vi "WriteSpreadsheet.vi"(0 "2-d array of\nnumbers":dbl[][](array[numeric])) -> ()   [LabVIEW 2023]
doc: "This is a tool that was written to allow users the opportunity to preview the files before they save them into a spreadsheet. The precision can be input and the header can be setup prior to saving the data."
panel:
  in  "invert data":bool
  in  "cancel":bool
  in  "save":bool
  in  "header":string[][](table)=[["User Name", "", "", "", "", "", "", "", "", "", ""], ["Experimental Description", "", "", "", "", "", "", "", "", "", ""], ["Header A (units)", "Header B (u)", "Header C (u)", "Header D (u)", "", "", "", "", "", "", ""]]
  in  "precision":i16=6 caption="input the desired\ndata precision"
  out "spreadsheet":string[][](table)=[["Sunday, January 10, 2010", "", "", "", "", "", "", "", "", "", ""], ["User Name", "", "", "", "", "", "", "", "", "", ""], ["Experimental Description", "", "", "", "", "", "", "", "", "", ""], ["Header A (units)", "Header B (u)", "Header C (u)", "Header D (u)", "", "", "", "", "", "", ""], ["NaN", "NaN", "NaN", "NaN", "", "", "", "", "", "", ""], ["NaN", "NaN", "NaN", "NaN", "", "", "", "", "", "", ""], ["NaN", "NaN", "NaN", "NaN", "", "", "", "", "", "", ""]]
  # "Input File Information and Headers (editable)"
  # "Spread Sheet Viewer (not editable)"
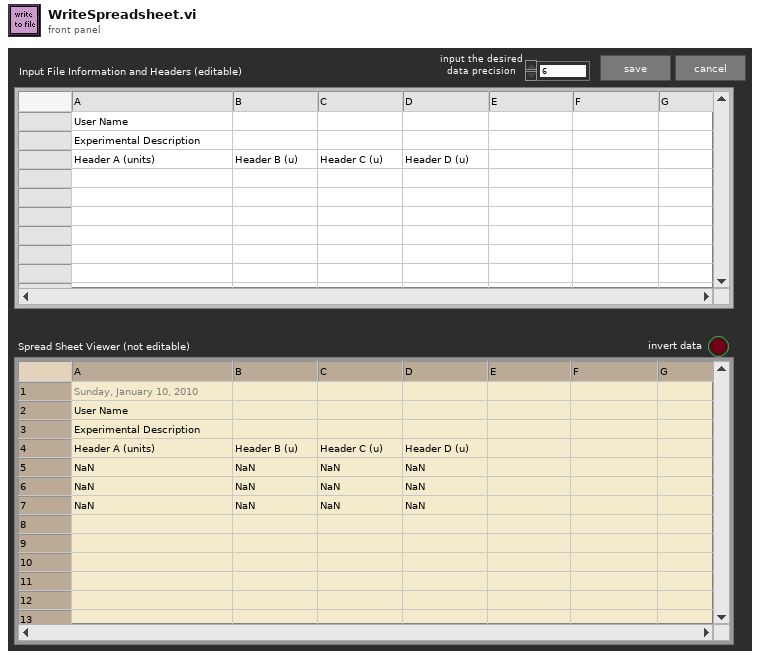
[diagram p1: front panel]
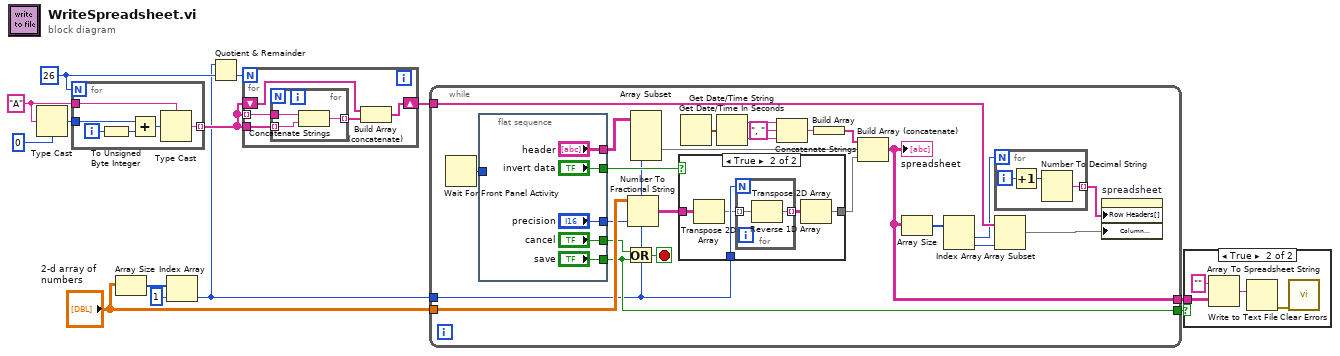
[diagram p0: block diagram]
diagram:
  w8 = 26
  w11 = "A" ("string")
  n1 = Type Cast(type=u8 0 ("element"), x=w11) -> (*(type *) &x=w9:u8)
  n2 = for {
    N: w8 -> [_]
    tunnel: w9 -> [w18]
    tunnel: [w14] -> w7 mode=indexing
    tunnel: w11 -> [w15]
    i -> [w19]
    n3 = To Unsigned Byte Integer(number=w19) -> (unsigned 8bit integer=w17:u8)
    n4 = Add(x=w18, y=w17) -> (x+y=w16:u8)
    n5 = Type Cast(type=w15, x=w16) -> (*(type *) &x=w14:string)
  }
  n6 = Array Size(array="2-d array of\nnumbers") -> (size(s)=w4:i32[])
  n7 = Index Array(array=w4, index=1) -> (element=w2:i32)
  n8 = Quotient & Remainder(x=w2, y=w8) -> (floor(x/y)=w6:i32)  [unwired: 1 out]
  n9 = for {
    N: w6 -> [_]
    tunnel: w7 -> [w24]
    tunnel: w7 -> [w23] mode=indexing
    shift-right: [w21] -> w5
    shift-left: w7 -> [w20]
    n10 = for {
      tunnel: w24 -> [w27] mode=indexing
      tunnel: w23 -> [w26]
      tunnel: [w25] -> w22 mode=indexing
      n11 = Concatenate Strings(w26, w27) -> (w25:string)
    }
    n12 = Build Array (concatenate)(w20, w22) -> (w21:string[])
  }
  n13 = while {
    tunnel: "2-d array of\nnumbers" -> [w44]
    tunnel: [w40] -> w13
    tunnel: [w39] -> w12
    tunnel: w5 -> [w47]
    tunnel: w2 -> [w28]
    stop <- w49 stop-if-true
    n14 = Wait For Front Panel Activity() -> (0:w42:u32)  [unwired: 3 in]
    n15 = flat-sequence {
      tunnel: w42 -> [_]
      tunnel: ["cancel"] -> w41
      tunnel: ["save"] -> w40
      tunnel: ["header"] -> w30
      tunnel: ["invert data"] -> w35
      tunnel: ["precision"] -> w34
      frame #0 {
      }
    }
    n16 = Or(x=w41, y=w40) -> (x .or. y?=w49:bool)
    n17 = Number To Fractional String(number=w44, precision (6)=w34) -> (F-format string=w43:string[][])  [unwired: 2 out]
    n18 = Array Subset(array=w30, length (col)=w28) -> (w29:string[][])  [unwired: 3 in]
    n19 = case shown="True" w35 {
      tunnel: w43 -> [w58 w62]
      tunnel: [w58 w59] -> w45
      tunnel: w28 -> [_ w63]
      frame False {
      }
      frame True {
        n20 = Transpose 2D Array(2D array=w62) -> (transposed array=w60:string[][])
        n21 = for {
          N: w63 -> [_]
          tunnel: w60 -> [w65] mode=indexing
          tunnel: [w64] -> w61 mode=indexing
          n22 = Reverse 1D Array(array=w65) -> (reversed array=w64:string[])
        }
        n23 = Transpose 2D Array(2D array=w61) -> (transposed array=w59:string[][])
      }
    }
    n24 = Get Date/Time In Seconds() -> (seconds since 1Jan1904=w52:timestamp)
    n25 = Get Date/Time String(seconds (now)=w52) -> (date string=w51:string, time string=w32:string)  [unwired: 1 in, 1 out]
    n26 = Concatenate Strings(w51, ", " ("string"), w32) -> (w50:string)
    n27 = Build Array(w50) -> (w33:string[])
    n28 = Build Array (concatenate)(w33, w29, w45) -> (w39:string[][])
    "spreadsheet" <- w39
    n29 = Array Size(array=w39) -> (size(s)=w48:i32[])
    n30 = Index Array(array=w48) -> (element #1=w38:i32, element #2=w37:i32)  [unwired: 2 in]
    n31 = for {
      N: w38 -> [_]
      tunnel: [w67] -> w46 mode=indexing
      i -> [w68]
      n32 = Increment(x=w68) -> (x+1=w66:i32)
      n33 = Number To Decimal String(number=w66) -> (decimal integer string=w67:string)  [unwired: 1 out]
    }
    n34 = Array Subset(array=w47, length=w37) -> (w36:string[])  [unwired: 1 in]
    n35 = property on="spreadsheet" class="Tbl (strict)"("Row Headers[]"=w46, "Column Headers[]"=w36) -> ()  [unwired: 2 in, 2 out]
  }
  n36 = case shown="True" w13 {
    tunnel: w12 -> [_ w71]
    frame False {
    }
    frame True {
      n37 = Array To Spreadsheet String(array=w71, 3:"" ("format string")) -> (spreadsheet string=w70:string)  [unwired: 1 in]
      n38 = Write to Text File(text=w70) -> (error out=w72:errorcluster)  [unwired: 1 in, 4 out]
      n39 = call <vilib>:"Clear Errors.vi"("error in (no error)"=w72) -> ()  [unwired: 1 in, 6 out]
    }
  }
